vi "solar_ui Listbox Initialize.vi"(10 "Selected Listbox Item":string, 11 "SOLAR":T1) -> (0 "Visible Target Names":string[](array[string]), 1 "Visible Targets":T2[](array[typedef]), 2 "TargetLB Symbols":i32[](array[numeric]), 3 "TargetLB Names":string[](array[string]), 4 "Selected Item Type":string, 6 "Relative Index of Item":i32)   [LabVIEW 2018]
doc: "This sets the SOLAR UI Target listbox items and symbols. The listbox is separated into Target, Voyager and QTimer sections. If <b>Selected Listbox Item</b> is set, this returns the <b>Selected Item Type</b> as 'TARGET', 'VOYAGER' or 'QTIMER' and returns the relative index of the item. If a target is hidden this does not add it to the listbox."
uses:
  solar_ctl Target Global.ctl
  voyager/solar_voy_ctl Voyager Refnum.ctl
  qtimer/solar_qtimer_ctl Refnum.ctl
  solar_ctl SOLAR Global.ctl
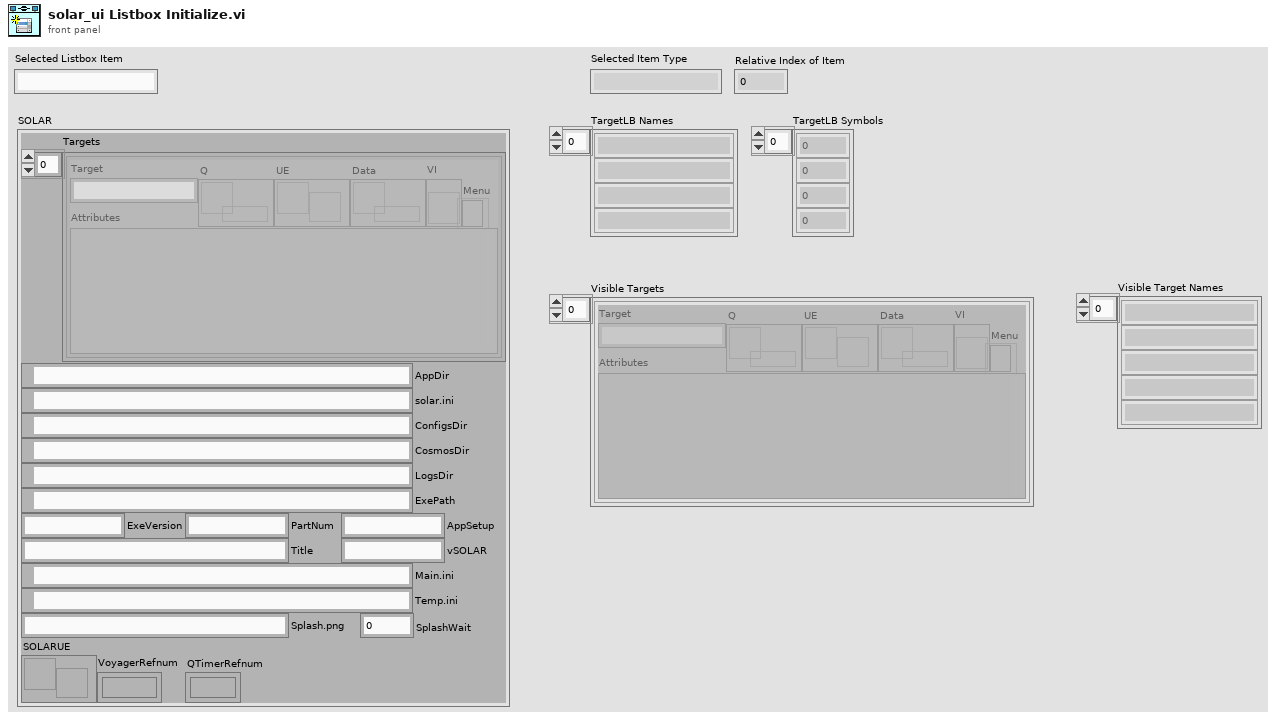
[diagram p1: front panel]
types:
  T1 = typedef "solar_ctl SOLAR Global.ctl" = cluster{"Targets":T2[], "AppDir":path, "solar.ini":path, "ConfigsDir":path, "CosmosDir":path, "LogsDir":path, "ExePath":path, "ExeVersion":string, "PartNum":string, "AppSetup":string, "Title":string, "Main.ini":path, "Temp.ini":path, "vSOLAR":string, "Splash.png":string, "SplashWait":i32, "SOLARUE":refnum<user-event>, "VoyagerRefnum":T3, "QTimerRefnum":T4}
  T2 = typedef "solar_ctl Target Global.ctl" = cluster{"Target":string, "Q":refnum<queue>, "UE":refnum<user-event>, "VI":refnum<vi>, "Menu":refnum<k9>, "Data":refnum<data-value>, "Attributes":variant}
  T3 = typedef "solar_voy_ctl Voyager Refnum.ctl" = refnum<k1>
  T4 = typedef "solar_qtimer_ctl Refnum.ctl" = refnum<k1>
  T5 = typedef "solar_qtimer_ctl QTimer.ctl" = cluster{"Settings":T6, "Queue":refnum<queue>, "QTimerQ":refnum<queue>, "VI Refnum":refnum<vi>}
  T6 = typedef "solar_qtimer_ctl QTimer Settings.ctl" = cluster{"QTimer":string, "Delay":i32, "Start":bool, "EnQ_Type":enum8{"Normal", "Priority", "IgnoreIfExists"}, "Messages":cluster{"MSG":string, "DATA":variant}[]}
  T7 = typedef "solar_voy_ctl Voyager.ctl" = cluster{"PACKETS":T8[], "COSMOS_Root":path, "CMD_HDR":T13, "TLM_HDR":T13, "TCPs":T14[], "VoyagerIDOffset":cluster{"VoyagerIDOffset":u16[], "Target Names":string[]}}
  T8 = typedef "solar_voy_def_ctl PACKET.ctl" = cluster{"PACKET_ID":T9, "ENDIAN":enum8{"BIG", "LITTLE"}, "DESC":string, "HZRD":bool, "ITEMS":T10[], "NoExport":bool, "last_time":timestamp, "last_count":u32, "last_data":string}
  T9 = typedef "solar_voy_def_ctl PACKET_ID.ctl" = cluster{"ID":u16, "CMD":enum8{"CMD", "TLM"}, "TARGET":string, "PACKET":string}
  T10 = typedef "solar_voy_def_ctl ITEM.ctl" = cluster{"NAME":string, "OFFSET":i32, "SIZE":i32, "TYPE":T11, "EACH_SIZE":i32, "LVTYPE":T12, "MIN":dbl, "MAX":dbl, "DEFAULT":string, "DESC":string, "ID":bool, "MODIFIERS":variant, "last_value":variant}
  T11 = typedef "solar_voy_def_ctl ITEM TYPE.ctl" = enum8{"BLOCK", "INT", "UINT", "FLOAT", "STRING"}
  T12 = typedef "solar_type Item Type.ctl" = enum16{"NULL", "UNKNOWN", "CLUSTER", "I8", "I16", "I32", "I64", "U8", "U16", "U32", "U64", "U8_ENUM", "U16_ENUM", "U32_ENUM", "SGL", "DBL", "BOOLEAN", "STRING", "PATH", "VISA", "TAG", "TIME", "I8_1D", "I16_1D", "I32_1D", "I64_1D", "U8_1D", "U16_1D", "U32_1D", "U64_1D", "U8_ENUM_1D", "U16_ENUM_1D", "U32_ENUM_1D", "SGL_1D", "DBL_1D", "BOOLEAN_1D", "STRING_1D", "PATH_1D", "VISA_1D", "TAG_1D", "TIME_1D", "I8_2D", "I16_2D", "I32_2D", "I64_2D", "U8_2D", "U16_2D", "U32_2D", "U64_2D", "U8_ENUM_2D", "U16_ENUM_2D", "U32_ENUM_2D", "SGL_2D", "DBL_2D", "BOOLEAN_2D", "STRING_2D", "PATH_2D", "VISA_2D", "TAG_2D", "TIME_2D"}
  T13 = typedef "solar_voy_def_ctl HDR.ctl" = cluster{"ITEMS":T10[], "LENGTH_NAME":string, "LENGTH_VALUE_OFFSET":i32, "ID_NAME":string, "ENDIAN":enum8{"BIG", "LITTLE"}, "GUID_NAME":string, "DEFAULT_TARGET":string, "DEFAULT_PACKET":string, "DEFAULT_ERROR":string}
  T14 = typedef "solar_voy_ctl TCP.ctl" = cluster{"Connected":bool, "Port":u16, "Listener":refnum<k5>, "ServerIP":string, "TCP":refnum<k5>, "Setup":T15, "VIRefnum":refnum<vi>, "TARGETS_CMD":string[], "TARGETS_TLM":string[]}
  T15 = typedef "solar_voy_ctl Port Setup.ctl" = enum8{"SERVER", "CLIENT", "SERVER_CMD", "SERVER_TLM"}
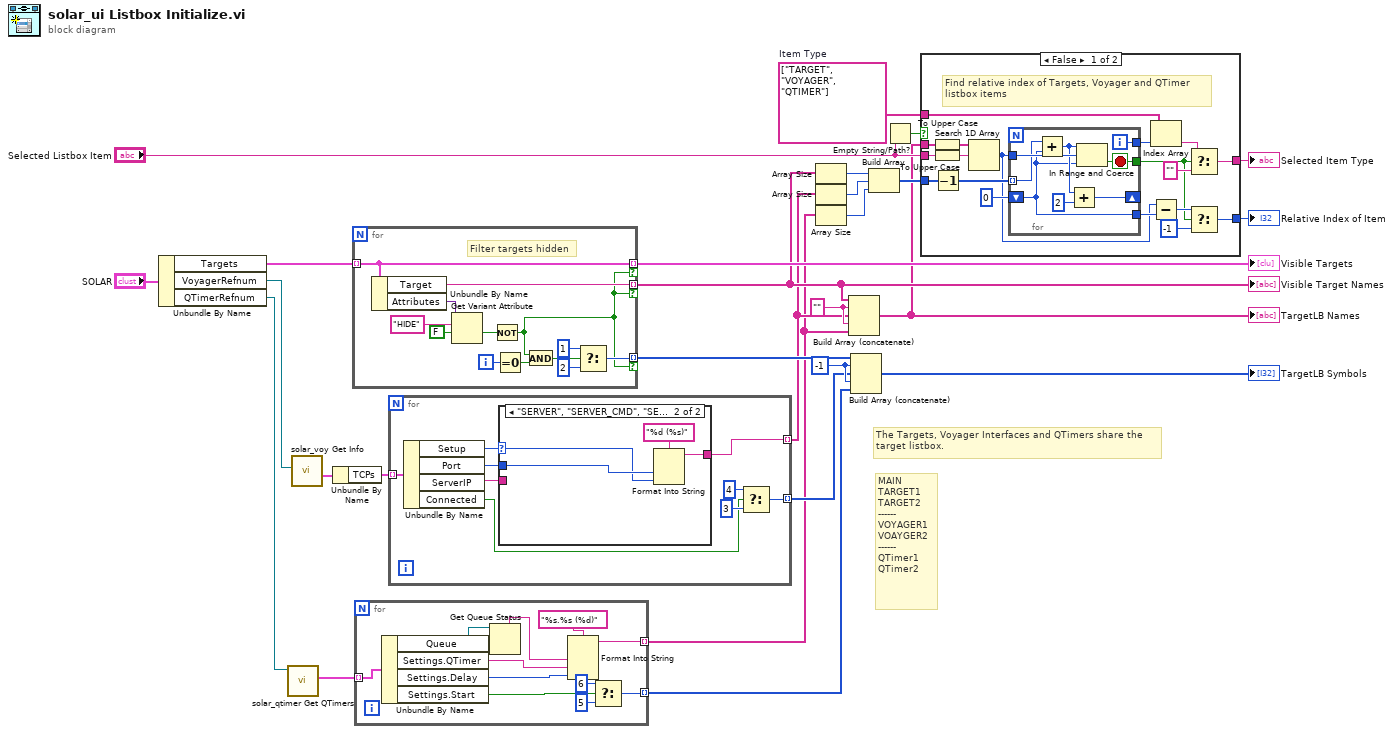
[diagram p0: block diagram]
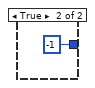
[diagram p2: hidden frame]
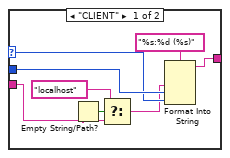
[diagram p3: hidden frame]
diagram:
  w11 = string[] ["TARGET", "VOYAGER", "QTIMER"]  # Item Type
  w26 = -1
  w25 = "" ("element")
  # "MAIN\nTARGET1\nTARGET2\n------\nVOYAGER1\nVOAYGER2\n------\nQTimer1\nQTimer2"
  # "The Targets, Voyager Interfaces and QTimers share the\ntarget listbox."
  n1 = Unbundle By Name("SOLAR") -> ("Targets"=w21:T2[], "VoyagerRefnum"=w18:T3, "QTimerRefnum"=w23:T4)
  n2 = call "solar_qtimer Get QTimers.vi"("QTimer Refnum"=w23) -> ("QTimers"=w24:T5[])  [unwired: 8 in, 2 out]
  n3 = call "solar_voy Get Info.vi"("Voyager Refnum"=w18) -> ("Voyager"=w19:T7)  [unwired: 8 in, 2 out]
  n4 = Unbundle By Name(w19) -> ("TCPs"=w20:T14[])
  n5 = for {
    tunnel: [w34] -> w7 mode=indexing if=w28
    tunnel: w21 -> [w29] mode=indexing
    tunnel: [w35] -> w14 mode=indexing if=w28
    tunnel: [w29] -> w22 mode=indexing if=w28
    i -> [w36]
    # "Filter targets hidden"
    n6 = Unbundle By Name(w29) -> ("Target"=w34:string, "Attributes"=w33:variant)
    n7 = Get Variant Attribute(Variant=w33, name="HIDE", default value (empty Variant)=FALSE) -> (value=w30:bool)  [unwired: 1 in, 3 out]
    n8 = Not(x=w30) -> (.not. x?=w28:bool)
    n9 = Equal To 0?(x=w36) -> (x = 0?=w38:bool)
    n10 = And(x=w28, y=w38) -> (x .and. y?=w37:bool)
    n11 = Select(t=1, s=w37, f=2) -> (s? t:f=w35:i32)
  }
  "Visible Targets" <- w22
  "Visible Target Names" <- w7
  n12 = for {
    tunnel: w24 -> [w51] mode=indexing
    tunnel: [w45] -> w5 mode=indexing
    tunnel: [w44] -> w27 mode=indexing
    n13 = Unbundle By Name(w51) -> ("Queue"=w43:refnum<queue>, "Settings.QTimer"=w42:string, "Settings.Delay"=w50:i32, "Settings.Start"=w46:bool)
    n14 = Get Queue Status(queue=w43) -> (queue name=w41:string)  [unwired: 2 in, 7 out]
    n15 = Format Into String(format string="%s.%s (%d)", w41, w42, w50) -> (resulting string=w45:string)  [unwired: 2 in, 1 out]
    n16 = Select(t=6, s=w46, f=5) -> (s? t:f=w44:i32)
  }
  n17 = for {
    tunnel: [w52] -> w6 mode=indexing
    tunnel: [w60] -> w17 mode=indexing
    tunnel: w20 -> [w57] mode=indexing
    n18 = Unbundle By Name(w57) -> ("Setup"=w56:T15, "Port"=w54:u16, "ServerIP"=w55:string, "Connected"=w53:bool)
    n19 = case shown="\"SERVER\", \"SERVER_CMD\", \"SERVER_TLM\"" w56 {
      selector: w56 -> [w65 w69]
      tunnel: [w68 w72] -> w52
      tunnel: w55 -> [w63 _]
      tunnel: w54 -> [w66 w70]
      frame "CLIENT" {
        n20 = Empty String/Path?(string/path=w63) -> (empty?=w64:bool)
        n21 = Select(t="localhost", s=w64, f=w63) -> (s? t:f=w62:string)
        n22 = Format Into String(format string="%s:%d (%s)", w62, w66, w65) -> (resulting string=w68:string)  [unwired: 2 in, 1 out]
      }
      frame "SERVER", "SERVER_CMD", "SERVER_TLM" {
        n23 = Format Into String(format string="%d (%s)", w70, w69) -> (resulting string=w72:string)  [unwired: 2 in, 1 out]
      }
    }
    n24 = Select(t=4, s=w53, f=3) -> (s? t:f=w60:i32)
  }
  n25 = Array Size(array=w7) -> (size(s)=w10:i32)
  n26 = Array Size(array=w6) -> (size(s)=w13:i32)
  n27 = Array Size(array=w5) -> (size(s)=w12:i32)
  n28 = Build Array (concatenate)(w7, w25, w6, w25, w5) -> (w1:string[])
  "TargetLB Names" <- w1
  n29 = Build Array (concatenate)(w14, w26, w17, w26, w27) -> (→"TargetLB Symbols":i32[])
  n30 = Build Array(w10, w13, w12) -> (w9:i32[])
  n31 = Empty String/Path?(string/path="Selected Listbox Item") -> (empty?=w8:bool)
  n32 = case shown="False" w8 {
    tunnel: "Selected Listbox Item" -> [w90 _]
    tunnel: [w84 _] -> w3
    tunnel: w11 -> [w83 _]
    tunnel: w1 -> [w73 _]
    tunnel: w9 -> [w82 _]
    tunnel: [w75 -1 ("f")] -> w2
    frame False {
      # "Find relative index of Targets, Voyager and QTimer\nlistbox items"
      n33 = To Upper Case(1:w73) -> (0:w74:string[])
      n34 = To Upper Case(1:w90) -> (0:w89:string)
      n35 = Decrement(x=w82) -> (x-1=w81:i32[])
      n36 = Search 1D Array(1D array=w74, element=w89) -> (index of element=w79:i32)  [unwired: 1 in]
      n37 = for {
        tunnel: w79 -> [w98]
        tunnel: w81 -> [w91] mode=indexing
        shift-right: [w95] -> _
        shift-left: 0 ("lower limit") -> [w92]
        tunnel: [w97] -> w87
        tunnel: [w96] -> w77
        tunnel: [w92] -> w80
        i -> [w97]
        stop <- w96 stop-if-true
        n38 = Add(x=w91, y=w92) -> (x+y=w93:i32)
        n39 = Add(x=w93, y=2) -> (x+y=w95:i32)
        n40 = In Range and Coerce(upper limit=w93, x=w98, lower limit=w92) -> (In Range?=w96:bool)  [unwired: 1 out]
      }
      n41 = Index Array(array=w83, index=w87) -> (element=w86:string)
      n42 = Subtract(x=w79, y=w80) -> (x-y=w78:i32)
      n43 = Select(t=w86, s=w77, f="") -> (s? t:f=w84:string)
      n44 = Select(t=w78, s=w77, f=-1) -> (s? t:f=w75:i32)
    }
    frame True {
    }
  }
  "Selected Item Type" <- w3
  "Relative Index of Item" <- w2
